vi "Endpoint Config Write.vi"(4 "error in (no error)":errorcluster, 5 "Value":T7[](array[typedef]), 6 "Container State":T10, 7 "Display State In":T1) -> (0 "error out":errorcluster, 3 "Display State Out":T1)   [LabVIEW 2020, in "Stimulus Channel (G3).xctl"]
uses:
  Stimulus Channel (G3).xctl
  <vilib>/_xctls/Container State.ctl
  Calibration VIs/Endpoint VIs/LV Source/Endpoint-Spec.ctl
  Calibration VIs/Endpoint VIs/LV Source/Endpoint-Modality.ctl
  Calibration VIs/Endpoint VIs/LV Source/Endpoint-Laterality.ctl
  State.ctl
  Burst (G3)/Controls.ctl
  Waveform XControls/Waveform (G3)/Waveform (G3).xctl
  Level (G3)/Level (G3).xctl
  Utility VIs/Controls/KRing/KRing.xctl
  Burst (G3)/Burst (G3).xctl
  Level (G3)/Level Units (G3).ctl
  Waveform VIs/Waveform Enum (V3).ctl
  Waveform XControls/Waveform (G3)/Waveform (G3) - Persistent.ctl
  Waveform XControls/Noise (G3)/Noise (G3) - Persistent.ctl
  <vilib>/_xctls/XControlSupport.lvlib
  Waveform XControls/Noise (G3)/Noise (G3).xctl
panel:
  # "Replace the Value Control below with a Control of desired type.\nDo not remove this Control or the others from the connector pane.\nDo not change the connector pane pattern.\nThe Value control should always be the third terminal from top on the input side in the connector pane."
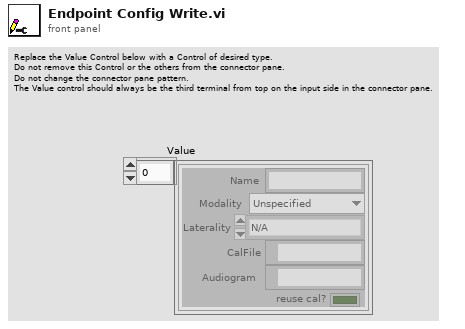
[diagram p1: front panel]
types:
  T1 = typedef "Stimulus Channel (G3).xctl/State.ctl" = cluster{"Show advanced":bool, "Show rove":bool, "Show name":bool, "Show dest":bool, "Lock dest":bool, "max level":dbl, "LMax Event":refnum<user-event>, "Controls":T2, "Level units":T3[], "Waveforms":T4[], "waveform":T5, "Endpoint Config":T7[], "multi":bool}
  T2 = typedef "Controls.ctl" = cluster{"Waveform":refnum<vi>, "Level":refnum<vi>, "Dest":refnum<vi>, "Gate":refnum<vi>}
  T3 = typedef "Level (G3).xctl/Level Units (G3).ctl" = enum16{"dB atten", "dB SPL", "dB re 1 Vrms", "dB V/Hz½", "mW", "dB HL", "Volts", "dB mW"}
  T4 = typedef "Waveform Enum (V3).ctl" = enum16{"OFF", "Tone", "Noise", "Pulse Train", "File", "FM Sweep", "Chirp Train", "Complex Tone", "FM Tone", "Vowel", "Ramp"}
  T5 = typedef "Waveform (G3).xctl/Waveform (G3) - Persistent.ctl" = cluster{"noise":T6, "Sort":bool}
  T6 = typedef "Noise (G3).xctl/Noise (G3) - Persistent.ctl" = cluster{"Show Aweight":bool}
  T7 = typedef "Endpoint-Spec.ctl" = cluster{"Name":string, "Modality":T8, "Laterality":T9, "CalFile":path, "Audiogram":path, "reuse cal?":bool}
  T8 = typedef "Endpoint-Modality.ctl" = enum16{"Unspecified", "Acoustic", "Electric", "Optical"}
  T9 = typedef "Endpoint-Laterality.ctl" = enum16{"N/A", "Right", "Left"}
  T10 = typedef "XControlSupport.lvlib/Container State.ctl" = cluster{"Indicator?":bool, "Run Mode?":bool, " Refnum":refnum<vi>}
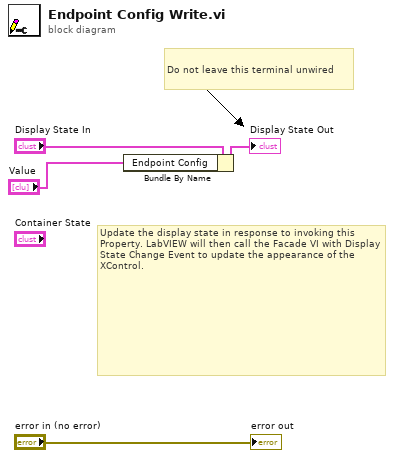
[diagram p0: block diagram]
diagram:
  # "Do not leave this terminal unwired"
  # "Update the display state in response to invoking this Property. LabVIEW will then call the Facade VI with Display State Change Event to update the appearance of the XControl."
  n1 = Bundle By Name(cluster="Display State In", "Endpoint Config"="Value") -> (→"Display State Out":T1)
  "error out" <- "error in (no error)"
